vi "Exc_1_2.vi"() -> ()   [LabVIEW 2016]
uses:
  <vilib>/DAQmx/read.llb/DAQmx Read (Digital Bool 1Line 1Point).vi
  <vilib>/DAQmx/write.llb/DAQmx Write (Digital Bool 1Line 1Point).vi
  <vilib>/DAQmx/create/channels.llb/DAQmx Create Channel (DI-Digital Input).vi
  <vilib>/DAQmx/create/channels.llb/DAQmx Create Channel (DO-Digital Output).vi
  <vilib>/DAQmx/miscellaneous.llb/DAQmx Fill In Error Info.vi
panel:
  out "Bottom Solenoid":bool
  out "Bottom Thing":bool
  out "Assemble Check":bool
  out "Bottom M":bool
  out "Dropper":bool
  out "Top Solenoid":bool
  out "Top Metal":bool
  out "Proximity Sensor":bool
  in  "Reject Solenoid":bool
  in  "Belt Motor":bool
  in  "Rotary":bool
  in  "Sort Solenoid":bool
  in  "Chain Motor":bool
  out "ICT_Stop":bool
  out "ICT_Start":bool
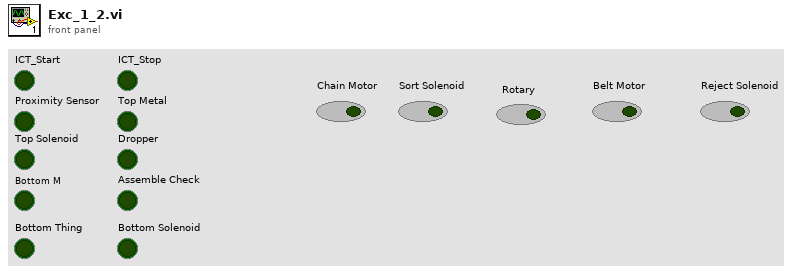
[diagram p1: front panel]
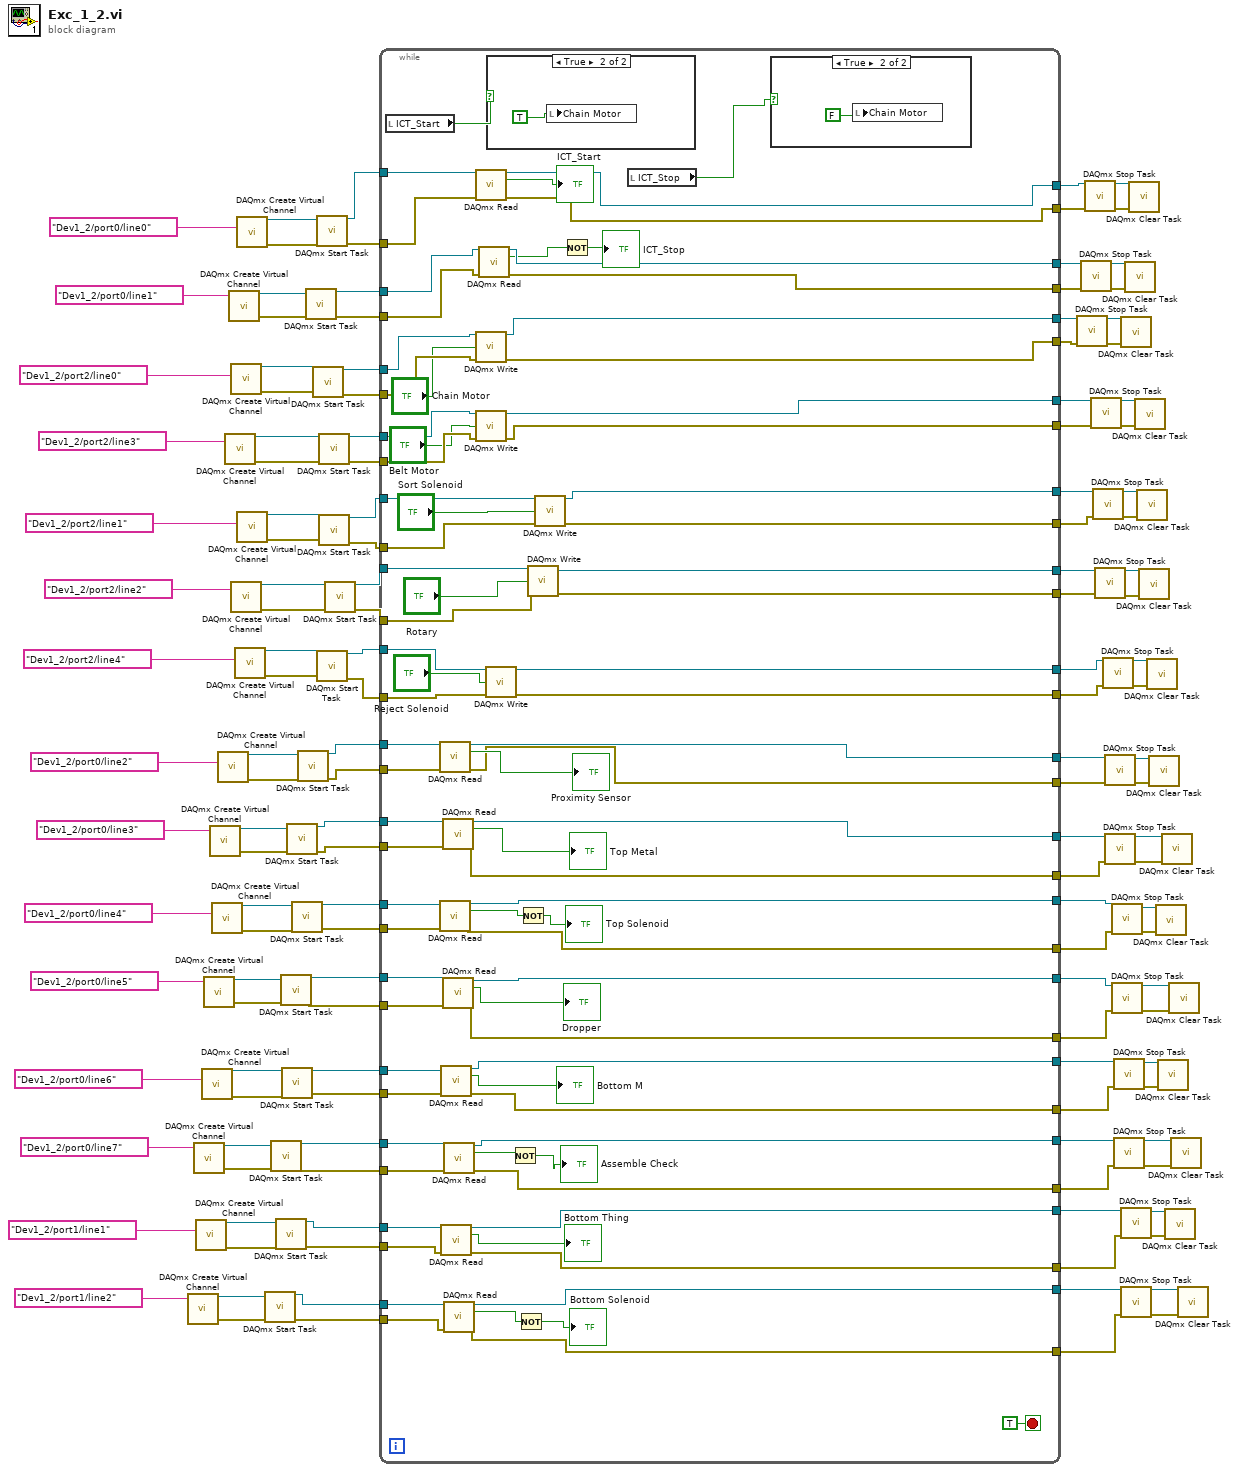
[diagram p0: block diagram]
diagram:
  n1 = call-poly <vilib>:"DAQmx Create Virtual Channel.vi"("lines"=tag "Dev1_2/port1/line2") -> ("task out"=w54:refnum<k21>, "error out"=w25:errorcluster)  [unwired: 13 in]
  n2 = call-poly <vilib>:"DAQmx Create Virtual Channel.vi"("lines"=tag "Dev1_2/port0/line7") -> ("task out"=w59:refnum<k21>, "error out"=w26:errorcluster)  [unwired: 13 in]
  n3 = call-poly <vilib>:"DAQmx Create Virtual Channel.vi"("lines"=tag "Dev1_2/port1/line1") -> ("task out"=w56:refnum<k21>, "error out"=w55:errorcluster)  [unwired: 13 in]
  n4 = call-poly <vilib>:"DAQmx Create Virtual Channel.vi"("lines"=tag "Dev1_2/port0/line6") -> ("task out"=w27:refnum<k21>, "error out"=w60:errorcluster)  [unwired: 13 in]
  n5 = call-poly <vilib>:"DAQmx Create Virtual Channel.vi"("lines"=tag "Dev1_2/port0/line5") -> ("task out"=w63:refnum<k21>, "error out"=w28:errorcluster)  [unwired: 13 in]
  n6 = call-poly <vilib>:"DAQmx Create Virtual Channel.vi"("lines"=tag "Dev1_2/port0/line3") -> ("task out"=w68:refnum<k21>, "error out"=w29:errorcluster)  [unwired: 13 in]
  n7 = call-poly <vilib>:"DAQmx Create Virtual Channel.vi"("lines"=tag "Dev1_2/port0/line4") -> ("task out"=w65:refnum<k21>, "error out"=w64:errorcluster)  [unwired: 13 in]
  n8 = call-poly <vilib>:"DAQmx Create Virtual Channel.vi"("lines"=tag "Dev1_2/port0/line2") -> ("task out"=w70:refnum<k21>, "error out"=w69:errorcluster)  [unwired: 13 in]
  n9 = call-poly <vilib>:"DAQmx Create Virtual Channel.vi"("lines"=tag "Dev1_2/port2/line3") -> ("task out"=w125:refnum<k21>, "error out"=w124:errorcluster)  [unwired: 13 in]
  n10 = call-poly <vilib>:"DAQmx Create Virtual Channel.vi"("lines"=tag "Dev1_2/port0/line1") -> ("task out"=w129:refnum<k21>, "error out"=w128:errorcluster)  [unwired: 13 in]
  n11 = call-poly <vilib>:"DAQmx Create Virtual Channel.vi"("lines"=tag "Dev1_2/port2/line0") -> ("task out"=w127:refnum<k21>, "error out"=w126:errorcluster)  [unwired: 13 in]
  n12 = call-poly <vilib>:"DAQmx Create Virtual Channel.vi"("lines"=tag "Dev1_2/port2/line2") -> ("task out"=w95:refnum<k21>, "error out"=w94:errorcluster)  [unwired: 13 in]
  n13 = call-poly <vilib>:"DAQmx Create Virtual Channel.vi"("lines"=tag "Dev1_2/port2/line4") -> ("task out"=w92:refnum<k21>, "error out"=w91:errorcluster)  [unwired: 13 in]
  n14 = call-poly <vilib>:"DAQmx Create Virtual Channel.vi"("lines"=tag "Dev1_2/port0/line0") -> ("task out"=w131:refnum<k21>, "error out"=w130:errorcluster)  [unwired: 13 in]
  n15 = call-poly <vilib>:"DAQmx Create Virtual Channel.vi"("lines"=tag "Dev1_2/port2/line1") -> ("task out"=w97:refnum<k21>, "error out"=w96:errorcluster)  [unwired: 13 in]
  n16 = call <vilib>:"DAQmx Start Task.vi"("task/channels in"=w54, "error in"=w25) -> ("task out"=w4:refnum<k21>, "error out"=w1:errorcluster)  [unwired: 12 in]
  n17 = call <vilib>:"DAQmx Start Task.vi"("task/channels in"=w59, "error in"=w26) -> ("task out"=w12:refnum<k21>, "error out"=w9:errorcluster)  [unwired: 12 in]
  n18 = call <vilib>:"DAQmx Start Task.vi"("task/channels in"=w56, "error in"=w55) -> ("task out"=w8:refnum<k21>, "error out"=w5:errorcluster)  [unwired: 12 in]
  n19 = call <vilib>:"DAQmx Start Task.vi"("task/channels in"=w63, "error in"=w28) -> ("task out"=w20:refnum<k21>, "error out"=w17:errorcluster)  [unwired: 12 in]
  n20 = call <vilib>:"DAQmx Start Task.vi"("task/channels in"=w27, "error in"=w60) -> ("task out"=w16:refnum<k21>, "error out"=w13:errorcluster)  [unwired: 12 in]
  n21 = call <vilib>:"DAQmx Start Task.vi"("task/channels in"=w68, "error in"=w29) -> ("task out"=w33:refnum<k21>, "error out"=w30:errorcluster)  [unwired: 12 in]
  n22 = call <vilib>:"DAQmx Start Task.vi"("task/channels in"=w65, "error in"=w64) -> ("task out"=w24:refnum<k21>, "error out"=w21:errorcluster)  [unwired: 12 in]
  n23 = call <vilib>:"DAQmx Start Task.vi"("task/channels in"=w70, "error in"=w69) -> ("task out"=w37:refnum<k21>, "error out"=w35:errorcluster)  [unwired: 12 in]
  n24 = call <vilib>:"DAQmx Start Task.vi"("task/channels in"=w129, "error in"=w128) -> ("task out"=w111:refnum<k21>, "error out"=w110:errorcluster)  [unwired: 12 in]
  n25 = call <vilib>:"DAQmx Start Task.vi"("task/channels in"=w127, "error in"=w126) -> ("task out"=w109:refnum<k21>, "error out"=w108:errorcluster)  [unwired: 12 in]
  n26 = call <vilib>:"DAQmx Start Task.vi"("task/channels in"=w131, "error in"=w130) -> ("task out"=w115:refnum<k21>, "error out"=w113:errorcluster)  [unwired: 12 in]
  n27 = call <vilib>:"DAQmx Start Task.vi"("task/channels in"=w92, "error in"=w91) -> ("task out"=w86:refnum<k21>, "error out"=w85:errorcluster)  [unwired: 12 in]
  n28 = call <vilib>:"DAQmx Start Task.vi"("task/channels in"=w125, "error in"=w124) -> ("task out"=w103:refnum<k21>, "error out"=w102:errorcluster)  [unwired: 12 in]
  n29 = call <vilib>:"DAQmx Start Task.vi"("task/channels in"=w97, "error in"=w96) -> ("task out"=w90:refnum<k21>, "error out"=w89:errorcluster)  [unwired: 12 in]
  n30 = call <vilib>:"DAQmx Start Task.vi"("task/channels in"=w95, "error in"=w94) -> ("task out"=w88:refnum<k21>, "error out"=w87:errorcluster)  [unwired: 12 in]
  n31 = while {
    tunnel: w115 -> [w214]
    tunnel: [w213] -> w114
    tunnel: w113 -> [w212]
    tunnel: [w211] -> w112
    tunnel: w111 -> [w210]
    tunnel: w110 -> [w209]
    tunnel: w109 -> [w208]
    tunnel: w108 -> [w207]
    tunnel: [w206] -> w107
    tunnel: [w205] -> w106
    tunnel: [w204] -> w105
    tunnel: [w203] -> w104
    tunnel: w103 -> [w202]
    tunnel: w102 -> [w201]
    tunnel: [w200] -> w101
    tunnel: [w199] -> w100
    tunnel: w90 -> [w193]
    tunnel: w89 -> [w192]
    tunnel: w88 -> [w191]
    tunnel: w87 -> [w190]
    tunnel: w86 -> [w189]
    tunnel: w85 -> [w188]
    tunnel: [w184] -> w78
    tunnel: [w183] -> w77
    tunnel: [w182] -> w76
    tunnel: [w181] -> w75
    tunnel: [w180] -> w74
    tunnel: [w179] -> w73
    tunnel: w37 -> [w173]
    tunnel: [w172] -> w36
    tunnel: w35 -> [w171]
    tunnel: [w170] -> w34
    tunnel: w33 -> [w169]
    tunnel: [w168] -> w32
    tunnel: [w167] -> w31
    tunnel: w30 -> [w166]
    tunnel: w24 -> [w165]
    tunnel: [w164] -> w23
    tunnel: [w163] -> w22
    tunnel: w21 -> [w162]
    tunnel: w20 -> [w161]
    tunnel: [w160] -> w19
    tunnel: [w159] -> w18
    tunnel: w17 -> [w158]
    tunnel: w16 -> [w157]
    tunnel: [w156] -> w15
    tunnel: [w155] -> w14
    tunnel: w13 -> [w154]
    tunnel: w12 -> [w153]
    tunnel: [w152] -> w11
    tunnel: [w151] -> w10
    tunnel: w9 -> [w150]
    tunnel: w8 -> [w149]
    tunnel: [w148] -> w7
    tunnel: [w147] -> w6
    tunnel: w5 -> [w146]
    tunnel: w4 -> [w145]
    tunnel: [w144] -> w3
    tunnel: [w143] -> w2
    tunnel: w1 -> [w142]
    stop <- TRUE stop-if-true
    n32 = local read "ICT_Start"() -> (w216:bool)
    n33 = call-poly <vilib>:"DAQmx Read.vi"("task/channels in"=w173, "error in"=w171) -> ("task out"=w172:refnum<k21>, "data"=→"Proximity Sensor":bool, "error out"=w170:errorcluster)  [unwired: 11 in]
    n34 = call-poly <vilib>:"DAQmx Read.vi"("task/channels in"=w165, "error in"=w162) -> ("task out"=w164:refnum<k21>, "data"=w136:bool, "error out"=w163:errorcluster)  [unwired: 11 in]
    n35 = call-poly <vilib>:"DAQmx Read.vi"("task/channels in"=w157, "error in"=w154) -> ("task out"=w156:refnum<k21>, "data"=→"Bottom M":bool, "error out"=w155:errorcluster)  [unwired: 11 in]
    n36 = call-poly <vilib>:"DAQmx Read.vi"("task/channels in"=w149, "error in"=w146) -> ("task out"=w148:refnum<k21>, "data"=→"Bottom Thing":bool, "error out"=w147:errorcluster)  [unwired: 11 in]
    n37 = call-poly <vilib>:"DAQmx Read.vi"("task/channels in"=w169, "error in"=w166) -> ("task out"=w168:refnum<k21>, "data"=→"Top Metal":bool, "error out"=w167:errorcluster)  [unwired: 11 in]
    n38 = call-poly <vilib>:"DAQmx Read.vi"("task/channels in"=w161, "error in"=w158) -> ("task out"=w160:refnum<k21>, "data"=→"Dropper":bool, "error out"=w159:errorcluster)  [unwired: 11 in]
    n39 = call-poly <vilib>:"DAQmx Read.vi"("task/channels in"=w153, "error in"=w150) -> ("task out"=w152:refnum<k21>, "data"=w139:bool, "error out"=w151:errorcluster)  [unwired: 11 in]
    n40 = call-poly <vilib>:"DAQmx Read.vi"("task/channels in"=w145, "error in"=w142) -> ("task out"=w144:refnum<k21>, "data"=w140:bool, "error out"=w143:errorcluster)  [unwired: 11 in]
    n41 = call-poly <vilib>:"DAQmx Read.vi"("task/channels in"=w214, "error in"=w212) -> ("task out"=w213:refnum<k21>, "data"=→"ICT_Start":bool, "error out"=w211:errorcluster)  [unwired: 11 in]
    n42 = call-poly <vilib>:"DAQmx Write.vi"("task/channels in"=w208, "data"="Chain Motor", "error in"=w207) -> ("task out"=w204:refnum<k21>, "error out"=w203:errorcluster)  [unwired: 10 in, 1 out]
    n43 = call-poly <vilib>:"DAQmx Write.vi"("task/channels in"=w202, "data"="Belt Motor", "error in"=w201) -> ("task out"=w200:refnum<k21>, "error out"=w199:errorcluster)  [unwired: 10 in, 1 out]
    n44 = call-poly <vilib>:"DAQmx Read.vi"("task/channels in"=w210, "error in"=w209) -> ("task out"=w206:refnum<k21>, "data"=w196:bool, "error out"=w205:errorcluster)  [unwired: 11 in]
    n45 = call-poly <vilib>:"DAQmx Write.vi"("task/channels in"=w189, "data"="Reject Solenoid", "error in"=w188) -> ("task out"=w180:refnum<k21>, "error out"=w179:errorcluster)  [unwired: 10 in, 1 out]
    n46 = case shown="True" w216 {
      frame False {
      }
      frame True {
        n47 = local write "Chain Motor"(TRUE) -> ()
      }
    }
    n48 = Not(x=w139) -> (.not. x?=→"Assemble Check":bool)
    n49 = Not(x=w140) -> (.not. x?=→"Bottom Solenoid":bool)
    n50 = Not(x=w136) -> (.not. x?=→"Top Solenoid":bool)
    n51 = call-poly <vilib>:"DAQmx Write.vi"("task/channels in"=w191, "data"="Rotary", "error in"=w190) -> ("task out"=w182:refnum<k21>, "error out"=w181:errorcluster)  [unwired: 10 in, 1 out]
    n52 = call-poly <vilib>:"DAQmx Write.vi"("task/channels in"=w193, "data"="Sort Solenoid", "error in"=w192) -> ("task out"=w184:refnum<k21>, "error out"=w183:errorcluster)  [unwired: 10 in, 1 out]
    n53 = Not(x=w196) -> (.not. x?=→"ICT_Stop":bool)
    n54 = local read "ICT_Stop"() -> (w215:bool)
    n55 = case shown="True" w215 {
      frame False {
      }
      frame True {
        n56 = local write "Chain Motor"(FALSE) -> ()
      }
    }
  }
  n57 = call <vilib>:"DAQmx Stop Task.vi"("task/channels in"=w105, "error in"=w104) -> ("task out"=w121:refnum<k21>, "error out"=w120:errorcluster)  [unwired: 12 in]
  n58 = call <vilib>:"DAQmx Stop Task.vi"("task/channels in"=w107, "error in"=w106) -> ("task out"=w119:refnum<k21>, "error out"=w118:errorcluster)  [unwired: 12 in]
  n59 = call <vilib>:"DAQmx Stop Task.vi"("task/channels in"=w114, "error in"=w112) -> ("task out"=w123:refnum<k21>, "error out"=w122:errorcluster)  [unwired: 12 in]
  n60 = call <vilib>:"DAQmx Stop Task.vi"("task/channels in"=w101, "error in"=w100) -> ("task out"=w117:refnum<k21>, "error out"=w116:errorcluster)  [unwired: 12 in]
  n61 = call <vilib>:"DAQmx Stop Task.vi"("task/channels in"=w78, "error in"=w77) -> ("task out"=w84:refnum<k21>, "error out"=w83:errorcluster)  [unwired: 12 in]
  n62 = call <vilib>:"DAQmx Stop Task.vi"("task/channels in"=w76, "error in"=w75) -> ("task out"=w80:refnum<k21>, "error out"=w79:errorcluster)  [unwired: 12 in]
  n63 = call <vilib>:"DAQmx Stop Task.vi"("task/channels in"=w74, "error in"=w73) -> ("task out"=w82:refnum<k21>, "error out"=w81:errorcluster)  [unwired: 12 in]
  n64 = call <vilib>:"DAQmx Stop Task.vi"("task/channels in"=w36, "error in"=w34) -> ("task out"=w47:refnum<k21>, "error out"=w51:errorcluster)  [unwired: 12 in]
  n65 = call <vilib>:"DAQmx Stop Task.vi"("task/channels in"=w32, "error in"=w31) -> ("task out"=w53:refnum<k21>, "error out"=w52:errorcluster)  [unwired: 12 in]
  n66 = call <vilib>:"DAQmx Stop Task.vi"("task/channels in"=w23, "error in"=w22) -> ("task out"=w46:refnum<k21>, "error out"=w48:errorcluster)  [unwired: 12 in]
  n67 = call <vilib>:"DAQmx Stop Task.vi"("task/channels in"=w19, "error in"=w18) -> ("task out"=w50:refnum<k21>, "error out"=w49:errorcluster)  [unwired: 12 in]
  n68 = call <vilib>:"DAQmx Stop Task.vi"("task/channels in"=w15, "error in"=w14) -> ("task out"=w39:refnum<k21>, "error out"=w43:errorcluster)  [unwired: 12 in]
  n69 = call <vilib>:"DAQmx Stop Task.vi"("task/channels in"=w11, "error in"=w10) -> ("task out"=w45:refnum<k21>, "error out"=w44:errorcluster)  [unwired: 12 in]
  n70 = call <vilib>:"DAQmx Clear Task.vi"("task in"=w121, "error in"=w120) -> ()  [unwired: 13 in, 1 out]
  n71 = call <vilib>:"DAQmx Stop Task.vi"("task/channels in"=w7, "error in"=w6) -> ("task out"=w38:refnum<k21>, "error out"=w40:errorcluster)  [unwired: 12 in]
  n72 = call <vilib>:"DAQmx Stop Task.vi"("task/channels in"=w3, "error in"=w2) -> ("task out"=w42:refnum<k21>, "error out"=w41:errorcluster)  [unwired: 12 in]
  n73 = call <vilib>:"DAQmx Clear Task.vi"("task in"=w119, "error in"=w118) -> ()  [unwired: 13 in, 1 out]
  n74 = call <vilib>:"DAQmx Clear Task.vi"("task in"=w123, "error in"=w122) -> ()  [unwired: 13 in, 1 out]
  n75 = call <vilib>:"DAQmx Clear Task.vi"("task in"=w117, "error in"=w116) -> ()  [unwired: 13 in, 1 out]
  n76 = call <vilib>:"DAQmx Clear Task.vi"("task in"=w84, "error in"=w83) -> ()  [unwired: 13 in, 1 out]
  n77 = call <vilib>:"DAQmx Clear Task.vi"("task in"=w80, "error in"=w79) -> ()  [unwired: 13 in, 1 out]
  n78 = call <vilib>:"DAQmx Clear Task.vi"("task in"=w82, "error in"=w81) -> ()  [unwired: 13 in, 1 out]
  n79 = call <vilib>:"DAQmx Clear Task.vi"("task in"=w47, "error in"=w51) -> ()  [unwired: 13 in, 1 out]
  n80 = call <vilib>:"DAQmx Clear Task.vi"("task in"=w46, "error in"=w48) -> ()  [unwired: 13 in, 1 out]
  n81 = call <vilib>:"DAQmx Clear Task.vi"("task in"=w39, "error in"=w43) -> ()  [unwired: 13 in, 1 out]
  n82 = call <vilib>:"DAQmx Clear Task.vi"("task in"=w53, "error in"=w52) -> ()  [unwired: 13 in, 1 out]
  n83 = call <vilib>:"DAQmx Clear Task.vi"("task in"=w38, "error in"=w40) -> ()  [unwired: 13 in, 1 out]
  n84 = call <vilib>:"DAQmx Clear Task.vi"("task in"=w50, "error in"=w49) -> ()  [unwired: 13 in, 1 out]
  n85 = call <vilib>:"DAQmx Clear Task.vi"("task in"=w45, "error in"=w44) -> ()  [unwired: 13 in, 1 out]
  n86 = call <vilib>:"DAQmx Clear Task.vi"("task in"=w42, "error in"=w41) -> ()  [unwired: 13 in, 1 out]
